vi "Camera Acquisition.vi"() -> ()   [LabVIEW 2014]
uses:
  SubVIs/Initilize Globals.vi
  lib/Andorlib/atmcd32d.lvlib
panel:
  out "Error Out 2":errorcluster
  in  "Stop Acquisition":bool=TRUE
  out "Andor Status":i32
  in  "Start Acquisiton?":bool=TRUE
  in  "Acquisition Parameters":T1
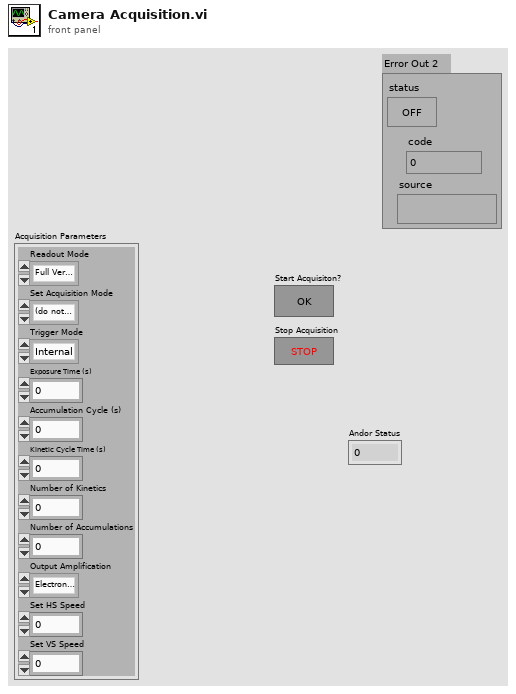
[diagram p1: front panel]
types:
  T1 = cluster{"Readout Mode":enum16{"Full Vertical Binning", "Multi-Track", "Random-Track", "Single-Track", "Image"}, "Set Acquisition Mode":enum16{"(do nothing)", "Single Scan", "Accumulate", "Kinetics", "Fast Kinetics", "Run till abort"}, "Trigger Mode":enum16{"Internal", "External"}, "Exposure Time (s)":dbl, "Accumulation Cycle (s)":dbl, "Kinetic Cycle Time (s)":dbl, "Number of Kinetics":i32, "Number of Accumulations":i32, "Output Amplification":enum16{"Electron Multiplication", "Extended NIR Mode"}, "Set HS Speed":i32, "Set VS Speed":i32}
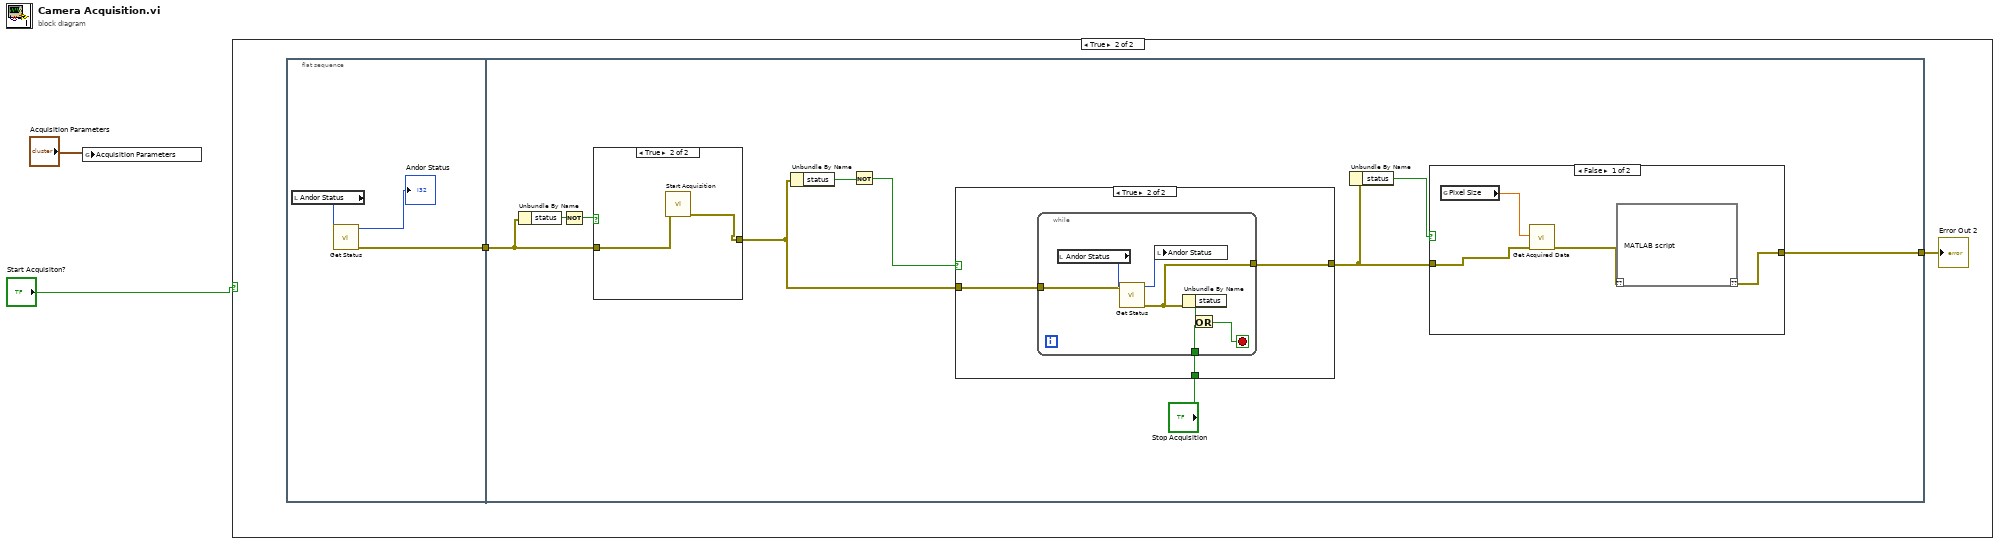
[diagram p0: block diagram]
diagram:
  n1 = global write "Initilize Globals.vi" "Acquisition Parameters"("Acquisition Parameters") -> ()
  n2 = case shown="True" "Start Acquisiton?" {
    frame False {
    }
    frame True {
      n3 = flat-sequence {
        tunnel: [w5] -> w4
        tunnel: w4 -> [w15]
        tunnel: [w8] -> w3
        frame #0 {
          n4 = local read "Andor Status"() -> (w6:i32)
          n5 = call "Get Status.vi"("status"=w6) -> ("error out"=w5:errorcluster, "status out"=→"Andor Status":i32)  [unwired: 8 in, 1 out]
        }
        frame #1 {
          n6 = Unbundle By Name(w15) -> ("status"=w16:bool)
          n7 = Not(x=w16) -> (.not. x?=w17:bool)
          n8 = case shown="True" w17 {
            tunnel: w15 -> [w34 w36]
            tunnel: [w34 w35] -> w12
            frame False {
            }
            frame True {
              n9 = call "Start Acquisition.vi"("error in (no error)"=w36) -> ("error out"=w35:errorcluster)  [unwired: 9 in, 1 out]
            }
          }
          n10 = Unbundle By Name(w12) -> ("status"=w14:bool)
          n11 = Not(x=w14) -> (.not. x?=w13:bool)
          n12 = case shown="True" w13 {
            tunnel: w12 -> [w23 w26]
            tunnel: [w23 w25] -> w9
            tunnel: "Stop Acquisition" -> [_ w24]
            frame False {
            }
            frame True {
              n13 = while {
                tunnel: w26 -> [w31]
                tunnel: [w30] -> w25
                tunnel: w24 -> [w28]
                stop <- w27 stop-if-true
                n14 = local read "Andor Status"() -> (w32:i32)
                n15 = call "Get Status.vi"("error in (no error)"=w31, "status"=w32) -> ("error out"=w30:errorcluster, "status out"=w33:i32)  [unwired: 7 in, 1 out]
                n16 = local write "Andor Status"(w33) -> ()
                n17 = Unbundle By Name(w30) -> ("status"=w29:bool)
                n18 = Or(x=w29, y=w28) -> (x .or. y?=w27:bool)
              }
            }
          }
          n19 = Unbundle By Name(w9) -> ("status"=w10:bool)
          n20 = case shown="False" w10 {
            tunnel: w9 -> [w20 w22]
            tunnel: [w18 w22] -> w8
            frame False {
              n21 = global read "Initilize Globals.vi" "Pixel Size"() -> (w21:dbl)
              n22 = call "Get Acquired Data.vi"("error in (no error)"=w20, "size"=w21) -> ("error out"=w19:errorcluster)  [unwired: 7 in, 2 out]
              n23 = script code="MATLAB script"("??"=w19) -> ("??"=w18:errorcluster)
            }
            frame True {
            }
          }
        }
      }
      "Error Out 2" <- w3
    }
  }
